vi "Config.vi"(8 "error in (no error)":errorcluster, 10 "Setting":T1={"dc voltage"=100, "high limit"=4e-07, "test time(s)"=3.0, "Channel"=""} {"high limit" format="%#_10f"}, 11 "HiPOT in":refnum<class "HiPOT.lvclass">) -> (0 "error out":errorcluster, 3 "HiPOT out":refnum<class "HiPOT.lvclass">)   [LabVIEW 2021, in "HAL.lvlib" / "HiPOT.lvclass"]
uses:
  HiPOT.lvclass
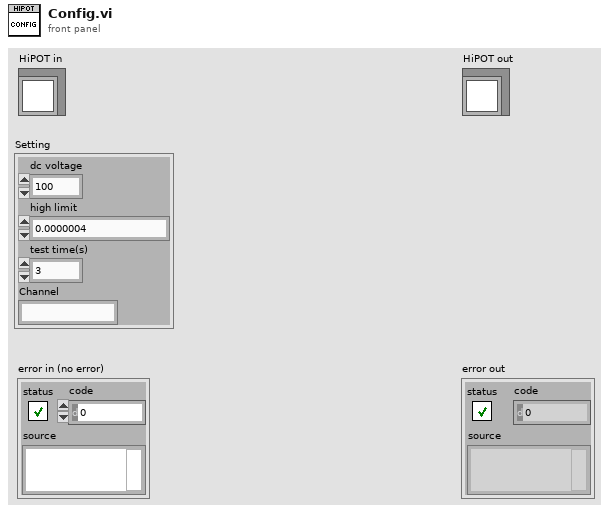
[diagram p1: front panel]
types:
  T1 = cluster{"dc voltage":i32, "high limit":dbl, "test time(s)":dbl, "Channel":string}
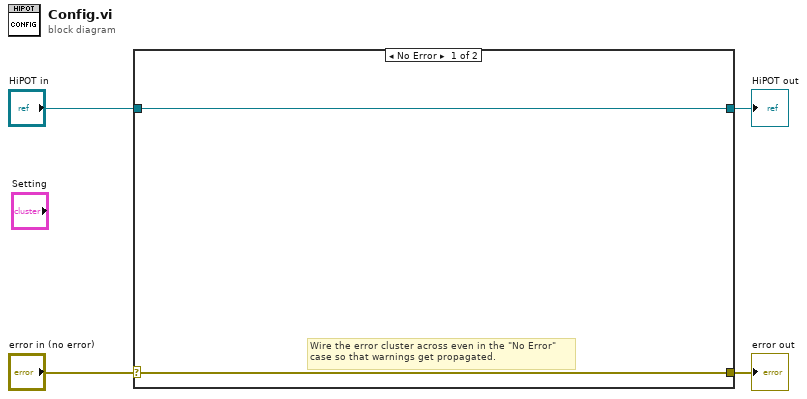
[diagram p0: block diagram]
diagram:
  n1 = case shown="No Error" "error in (no error)" {
    selector: "error in (no error)" -> [w5 w8]
    tunnel: [w5 w8] -> w3
    tunnel: [w6 w7] -> w1
    tunnel: "HiPOT in" -> [w6 w7]
    frame No Error {
      # "Wire the error cluster across even in the \"No Error\"\ncase so that warnings get propagated."
    }
    frame Error {
    }
  }
  "error out" <- w3
  "HiPOT out" <- w1
